vi "DAQmx Create Channel (AI-Pressure-Bridge-Two-Point-Linear).vi"(0 "task in":refnum<k21>, 1 "maximum value":dbl=100.0 format="%0.2f", 2 "minimum value":dbl=-100.0 format="%0.2f", 3 "bridge information":T1={"bridge configuration"=10182, "voltage excitation source"=10200, "voltage excitation value"=2.5, "nominal bridge resistance"=350.0} {"voltage excitation source" items=["Internal"=10200, "External"=10167]; "bridge configuration" items=["Full Bridge"=10182, "Half Bridge"=10187, "Quarter Bridge"=10270]}, 5 "physical channels":tag, 7 "name to assign":string, 9 "units":i32(ring)=15879 items=["Pascals"=10081, "psi"=15879, "bar"=15880, "From Custom Scale"=10065], 11 "error in":errorcluster, 12 "custom scale name":tag, 14 "scaling information":T2={"first electrical value"=0.0, "second electrical value"=2.0, "electrical units"=15897, "first physical value"=0.0, "second physical value"=100.0, "physical units"=15879} {"physical units" items=["Pascals"=10081, "psi"=15879, "bar"=15880]; "electrical units" items=["Volts/Volt"=15896, "mVolts/Volt"=15897]}) -> (4 "task out":refnum<k21>, 15 "error out":errorcluster)   [LabVIEW 2013]
doc: "Creates channel(s) that use a Wheatstone bridge to measure pressure. Use this instance with sensors whose specifications do not provide a polynomial for scaling or a table of electrical and physical values. When you use this scaling type, NI-DAQmx uses two points of electrical and physical values to calculate the slope and y-intercept of a linear equation and uses that equation to scale electrical values to physical values."
uses:
  <resource>/objmgr/daqmx.rc
panel:
  # "input limits"
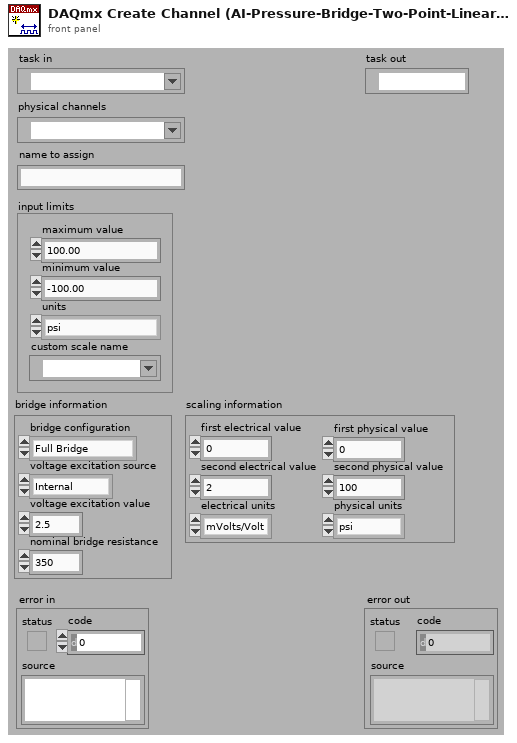
[diagram p1: front panel]
types:
  T1 = cluster{"bridge configuration":i32, "voltage excitation source":i32, "voltage excitation value":dbl, "nominal bridge resistance":dbl}
  T2 = cluster{"first electrical value":dbl, "second electrical value":dbl, "electrical units":i32, "first physical value":dbl, "second physical value":dbl, "physical units":i32}
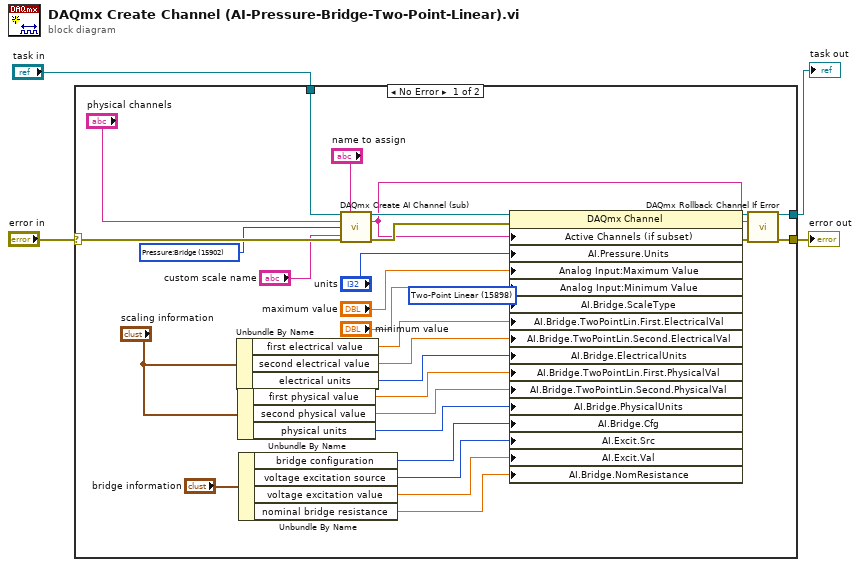
[diagram p0: block diagram]
diagram:
  n1 = case shown="No Error" "error in" {
    selector: "error in" -> [w32 w34]
    tunnel: [w24 w34] -> w4
    tunnel: "task in" -> [w33 w35]
    tunnel: [w23 w35] -> w1
    frame No Error {
      w5 = 15902 items=["Voltage"=10322, "Voltage RMS"=10350, "Current"=10134, "Current RMS"=10351, "More:Voltage:Custom with Excitation"=10323, "More:Bridge (V/V)"=15908, "Frequency"=10181, "Resistance"=10278, "Temperature:Thermocouple"=10303, "Temperature:Thermistor"=10302, "Temperature:RTD"=10301, "Temperature:Built-in Sensor"=10311, "Strain Gage"=10300, "Position:LVDT"=10352, "Position:RVDT"=10353, "Position:Eddy Current Proximity Probe"=14835, "Accelerometer"=10356, "Force:Bridge"=15899, "Force:IEPE Sensor"=15895, "Pressure:Bridge"=15902, "Sound Pressure:Microphone"=10354, "Torque:Bridge"=15905, "TEDS Sensor"=12531] ("AI.MeasType")
      w7 = 15898 items=["None"=10230, "Two-Point Linear"=15898, "Table"=10450, "Polynomial"=10449] ("AI.Bridge.ScaleType")
      n2 = Unbundle By Name("scaling information") -> ("first electrical value"=w18:dbl, "second electrical value"=w17:dbl, "electrical units"=w16:i32)
      n3 = Unbundle By Name("scaling information") -> ("first physical value"=w15:dbl, "second physical value"=w14:dbl, "physical units"=w13:i32)
      n4 = Unbundle By Name("bridge information") -> ("bridge configuration"=w11:i32, "voltage excitation source"=w10:i32, "voltage excitation value"=w9:dbl, "nominal bridge resistance"=w8:dbl)
      n5 = call "DAQmx Create AI Channel (sub).vi"("task in"=w33, "virtual channel name"="name to assign", "physical channel name"="physical channels", "measurement type"=w5, "error in"=w32, "custom scale"="custom scale name") -> ("task out"=w25:refnum<k21>, "channel names"=w22:string, "error out"=w30:errorcluster)  [unwired: 7 out]
      n6 = property class="DAQmx Channel"(reference=w25, error in=w30, "Active Channels (if subset)"=w22, "AI.Pressure.Units"="units", "Analog Input:Maximum Value"="maximum value", "Analog Input:Minimum Value"="minimum value", "AI.Bridge.ScaleType"=w7, "AI.Bridge.TwoPointLin.First.ElectricalVal"=w18, "AI.Bridge.TwoPointLin.Second.ElectricalVal"=w17, "AI.Bridge.ElectricalUnits"=w16, "AI.Bridge.TwoPointLin.First.PhysicalVal"=w15, "AI.Bridge.TwoPointLin.Second.PhysicalVal"=w14, "AI.Bridge.PhysicalUnits"=w13, "AI.Bridge.Cfg"=w11, "AI.Excit.Src"=w10, "AI.Excit.Val"=w9, "AI.Bridge.NomResistance"=w8) -> (reference out=w20:refnum<k21>, error out=w19:errorcluster)
      n7 = call "DAQmx Rollback Channel If Error.vi"("task in"=w20, "channel names"=w22, "error in"=w19) -> ("task out"=w23:refnum<k21>, "error out"=w24:errorcluster)  [unwired: 11 out]
    }
    frame Error {
    }
  }
  "error out" <- w4
  "task out" <- w1
